vi "KCubeActionEngine.vi"(5 "ChannelNumber":i32, 7 "Position Settings":T2={"Step Size (mm)"=10.0, "Initial Position"=0.0, "Num Of Steps"=200, "Move Position"=0.0, "Step Delay (ms)"=0} {"Step Size (mm)" min=0.00046 format="%.8f"}, 8 "SerialNumber":string="26004239", 9 "KCubeStepperControl":refnum<k24>(container), 10 "Action":T3) -> (0 "error out":errorcluster, 2 "Current Position":dbl)   [LabVIEW 2022 SP3]
uses:
  C:/Users/ulate/Documents/mnOP/mnOPSuite-main/PRISM/Thorlabs.MotionControl.Controls.dll
  mnOPSuite-main/PRISM/Thorlabs.MotionControl.Controls.dll
  ActionEngineEnum.ctl
  C:/Users/ulate/Documents/mnOP/mnOPSuite-main/PRISM/Thorlabs.MotionControl.KCube.StepperMotorCLI.dll
  mnOPSuite-main/PRISM/Thorlabs.MotionControl.KCube.StepperMotorCLI.dll
  C:/Users/ulate/Documents/mnOP/mnOPSuite-main/PRISM/Thorlabs.MotionControl.GenericMotorCLI.dll
  mnOPSuite-main/PRISM/Thorlabs.MotionControl.GenericMotorCLI.dll
panel:
  out "DeviceSettingsBasedOnName":string
  in  "startupSettingsMode":i32(ring)=1 items=["UseDeviceSettings"=1, "UseFileSettings"=2, "UseConfiguredSettings"=3]
  out "Settings":T1
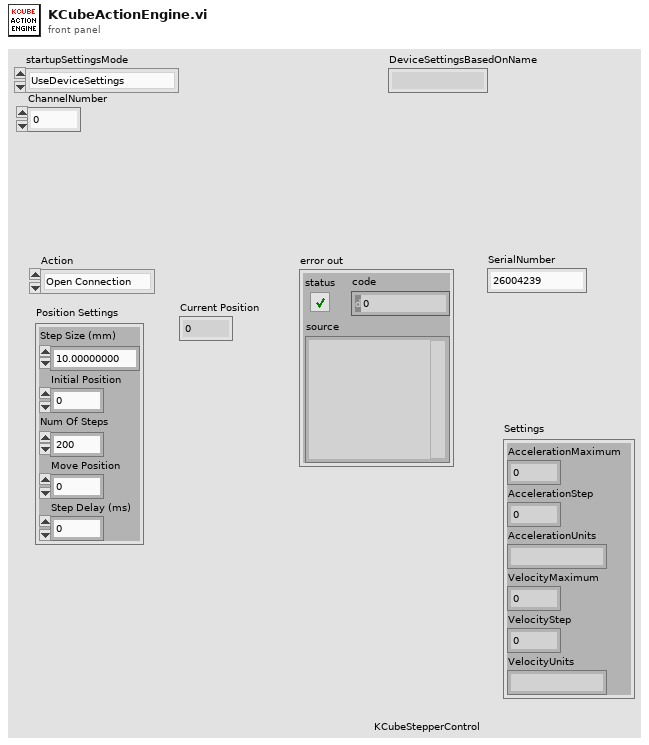
[diagram p1: front panel]
types:
  T1 = cluster{"AccelerationMaximum":dbl, "AccelerationStep":dbl, "AccelerationUnits":string, "VelocityMaximum":dbl, "VelocityStep":dbl, "VelocityUnits":string}
  T2 = cluster{"Step Size (mm)":sgl, "Initial Position":dbl, "Num Of Steps":i32, "Move Position":dbl, "Step Delay (ms)":u32}
  T3 = typedef "ActionEngineEnum.ctl" = enum16{"Open Connection", "Done", "Get Position", "Settings", "Home", "Move Absolute", "Move Relative", "Step", "Close Connection"}
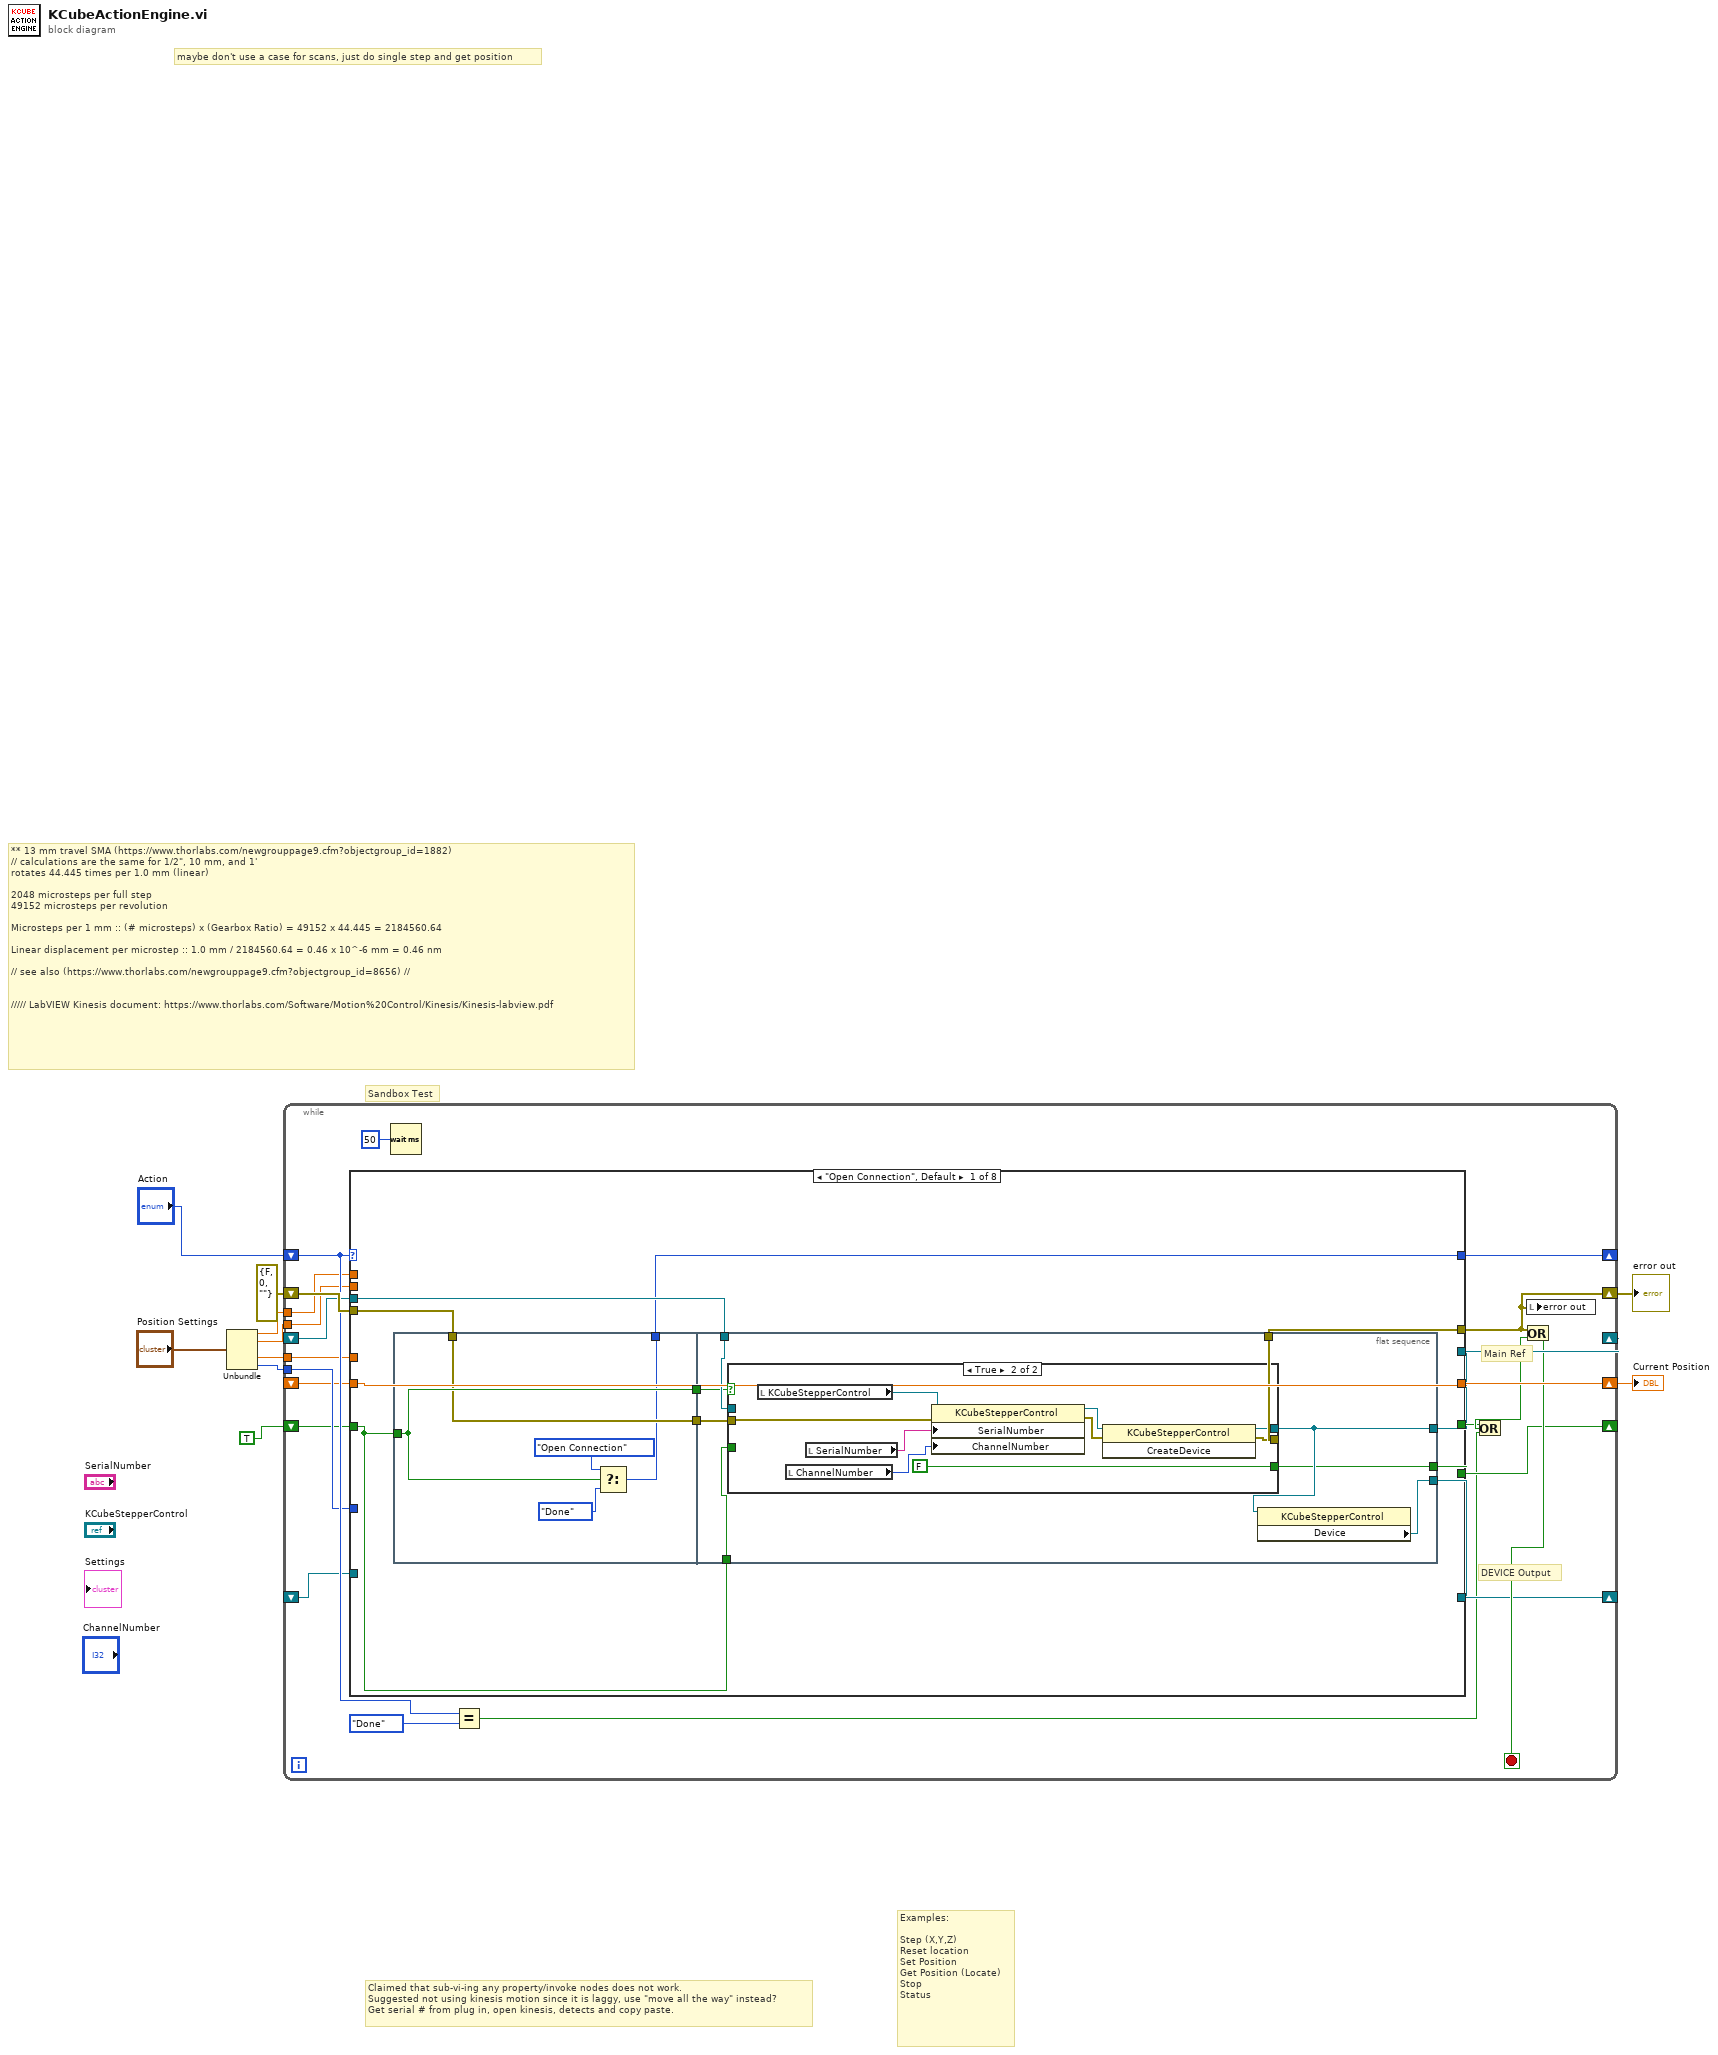
[diagram p0: block diagram]
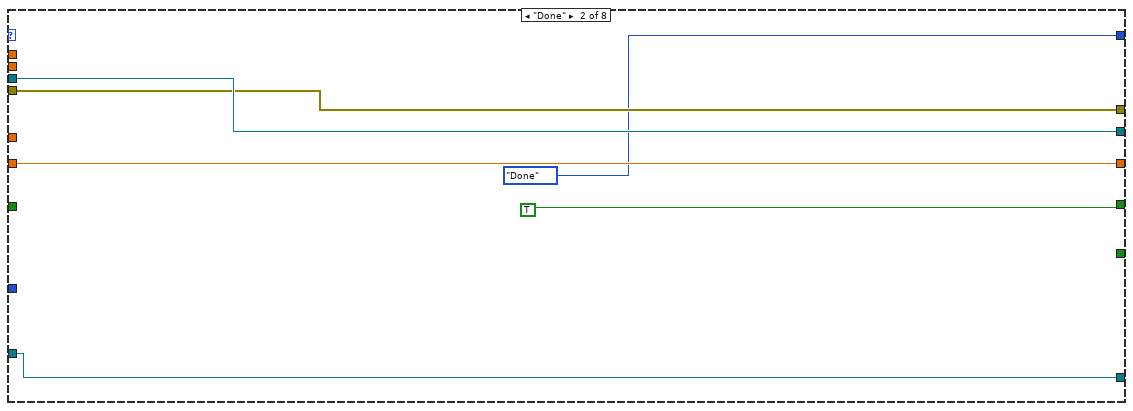
[diagram p3: hidden frame]
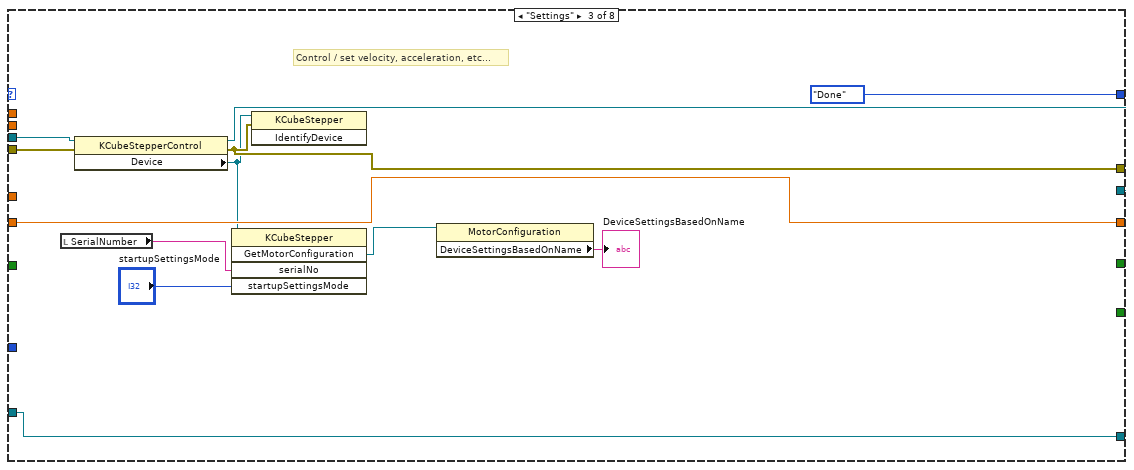
[diagram p4: hidden frame]
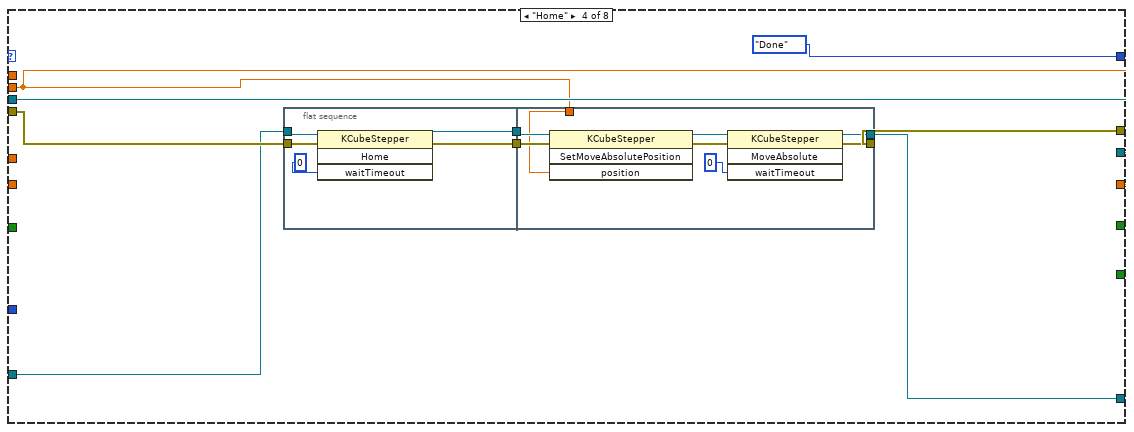
[diagram p5: hidden frame]
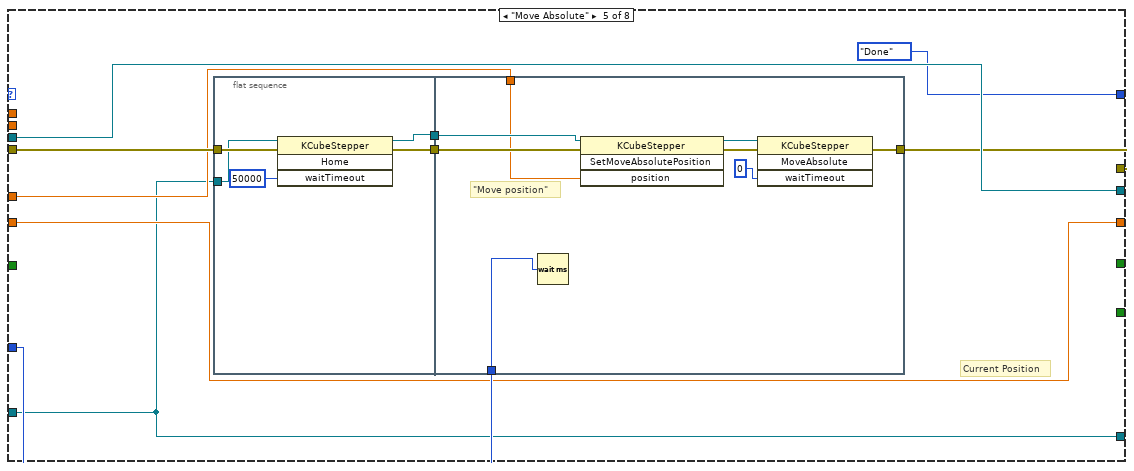
[diagram p6: hidden frame]
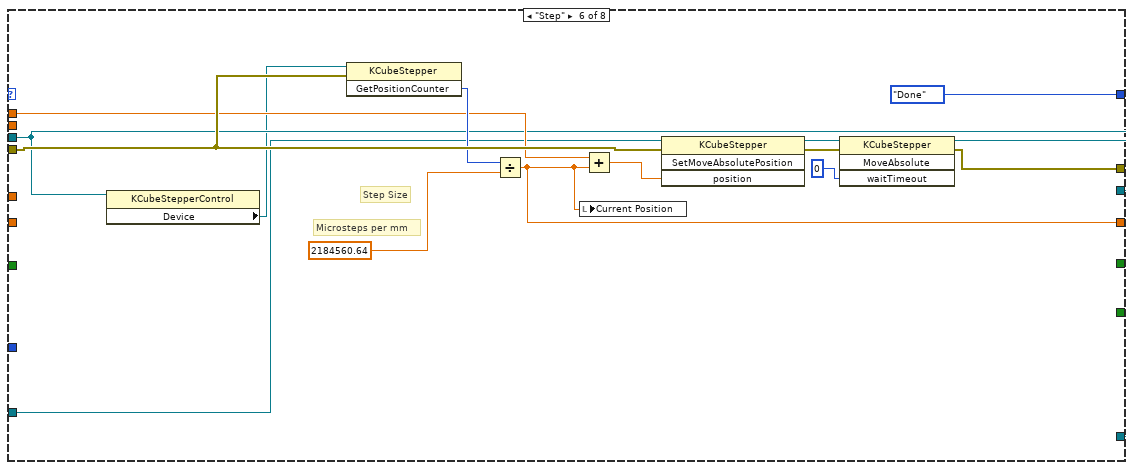
[diagram p7: hidden frame]
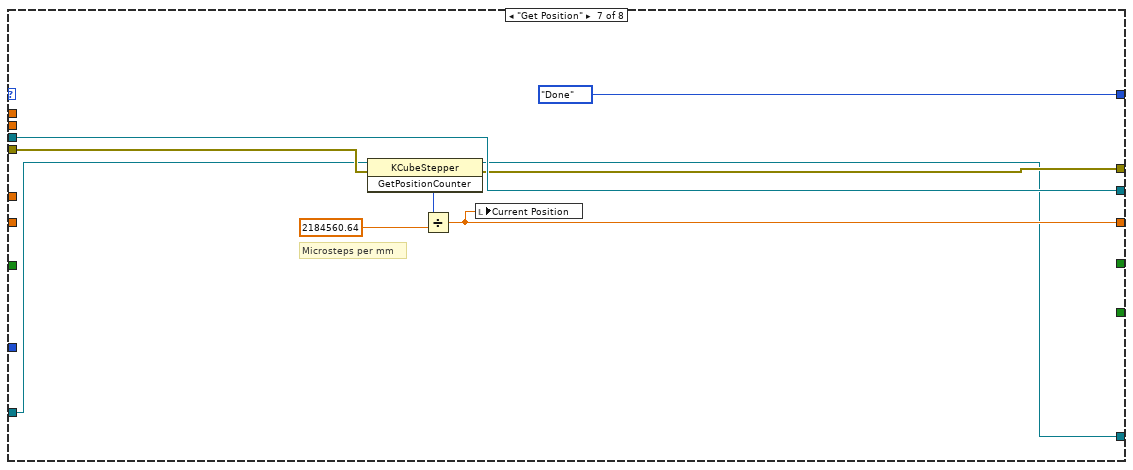
[diagram p8: hidden frame]
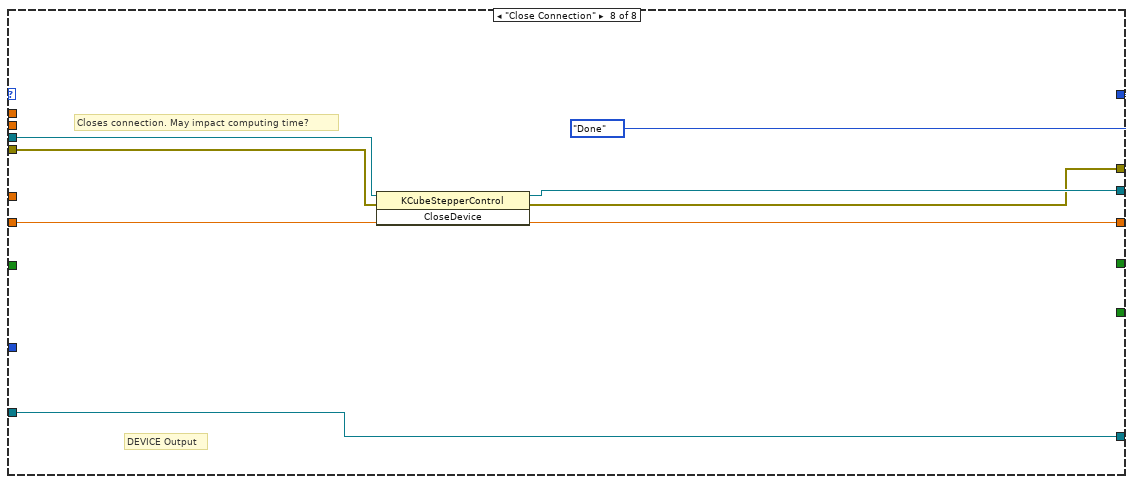
[diagram p9: hidden frame]
diagram:
  # "Claimed that sub-vi-ing any property/invoke nodes does not work.\nSuggested not using kinesis motion since it is laggy, use \"move all the way\" instead?\nGet serial # from plug in, open kinesis, detects and copy paste."
  # "maybe don't use a case for scans, just do single step and get position"
  # "Examples:\n\nStep (X,Y,Z)\nReset location\nSet Position\nGet Position (Locate) \nStop\nStatus"
  # "** 13 mm travel SMA (https://www.thorlabs.com/newgrouppage9.cfm?objectgroup_id=1882)\n// calculations are the same for 1/2\", 10 mm, and 1'\nrotates 44.445 times per 1.0 mm (linear)\n\n2048 microsteps per full step\n49152 microsteps per revolution\n\nMicrosteps per 1 mm :: (# microsteps) x (Gearbox Ratio) = 49152 x 44.445 = 2184560.64\n\nLinear displacement per microstep :: 1.0 mm / 2184560.64 = 0.46 x 10^-6 mm = 0.46 nm\n\n// see also (https://www.thorlabs.com/newgrouppage9.cfm?objectgroup_id=8656) //\n\n\n///// LabVIEW Kinesis document: https://www.thorlabs.com/Software/Motion%20Control/Kinesis/Kinesis-labview.pdf"
  # "Sandbox Test"
  n1 = Unbundle("Position Settings") -> ("Step Size (mm)"=w7:sgl, "Initial Position"=w8:dbl, "Move Position"=w5:dbl, "Step Delay (ms)"=w6:u32)  [unwired: 1 out]
  n2 = while {
    shift-right: [w19] -> w10
    shift-left: errorcluster {"status"=FALSE, "code"=0, "source"=""} ("error out") -> [w32]
    shift-right: [w30] -> _
    shift-left: _ -> [w31]
    shift-right: [w28] -> _
    shift-left: "Action" -> [w29]
    tunnel: w8 -> [w25]
    tunnel: w7 -> [w24]
    tunnel: w6 -> [w23]
    tunnel: w5 -> [w22]
    shift-right: [w21] -> w4
    shift-left: _ -> [w20]
    shift-right: [w17] -> _
    shift-left: _ -> [w16]
    shift-right: [w14] -> _
    shift-left: TRUE -> [w15]
    stop <- w18 stop-if-true
    # "DEVICE Output"
    # "Main Ref"
    n3 = case shown="\"Open Connection\", Default" w29 {
      tunnel: w32 -> [w42 w72 w84 w91 w118 w143 w154 w160]
      tunnel: [w39 w72 w81 w92 w110 w142 w151 w156] -> w19
      tunnel: w31 -> [w41 w73 w85 w95 w114 w133 w155 w158]
      tunnel: [w34 w73 w83 w95 w114 w133 w155 w157] -> w30
      tunnel: [w35 ActionEngineEnum."Done" ("Action") ActionEngineEnum."Done" ("Enum") ActionEngineEnum."Done" ("Enum") ActionEngineEnum."Done" ("Enum") ActionEngineEnum."Done" ("Enum") ActionEngineEnum."Done" ("Enum") ActionEngineEnum."Done" ("Enum")] -> w28
      tunnel: w25 -> [_ _ _ w90 _ _ _ _]
      tunnel: w24 -> [_ _ _ _ _ w138 _ _]
      tunnel: w23 -> [_ _ _ _ w115 _ _ _]
      tunnel: w22 -> [_ _ _ _ w113 _ _ _]
      tunnel: [w43 w74 w86 w90 w112 w137 w149 w161] -> w21
      tunnel: w20 -> [w43 w74 w86 _ w112 _ _ w161]
      tunnel: [w33 w71 w80 w88 w111 w135 w147 w159] -> w17
      tunnel: w16 -> [_ w71 w80 w89 w111 w134 w148 w159]
      tunnel: w15 -> [w40 _ _ _ _ _ _ _]
      tunnel: [w37 _ _ _ _ _ _ _] -> w14
      tunnel: [_ TRUE _ _ _ _ _ _] -> w11
      frame "Open Connection", Default {
        n4 = flat-sequence {
          tunnel: w40 -> [w48]
          tunnel: w42 -> [w45]
          tunnel: [w45] -> w38
          tunnel: [w48] -> w36
          tunnel: [w44] -> w35
          tunnel: w41 -> [w56]
          tunnel: w40 -> [w55]
          tunnel: [w49] -> w33
          tunnel: [w54] -> w39
          tunnel: [w52] -> w34
          tunnel: w38 -> [w53]
          tunnel: [w51] -> w37
          tunnel: w36 -> [w50]
          frame #0 {
            n5 = Select(t=ActionEngineEnum."Open Connection" ("Enum"), s=w48, f=ActionEngineEnum."Done" ("Enum")) -> (s? t:f=w44:T3)
          }
          frame #1 {
            n6 = case shown="True" w50 {
              selector: w50 -> [w57 _]
              tunnel: [w59 w66] -> w54
              tunnel: w53 -> [w59 w68]
              tunnel: [w58 w67] -> w52
              tunnel: w56 -> [w58 _]
              tunnel: w55 -> [_ _]
              tunnel: [w57 FALSE] -> w51
              frame False {
              }
              frame True {
                n7 = local read "KCubeStepperControl"() -> (w63:refnum<k24>)
                n8 = local read "ChannelNumber"() -> (w60:i32)
                n9 = local read "SerialNumber"() -> (w62:string)
                n10 = property class="KCubeStepperControl"(reference=w63, error in=w68, "SerialNumber"=w62, "ChannelNumber"=w60) -> (reference out=w65:refnum<k24>, error out=w64:errorcluster)
                n11 = invoke class="KCubeStepperControl" method="CreateDevice"(reference=w65, error in=w64) -> (reference out=w67:refnum<k24>, error out=w66:errorcluster)  [unwired: 1 in, 1 out]
              }
            }
            n12 = property class="KCubeStepperControl"(reference=w52) -> ("Device"=w49:refnum<k24>)  [unwired: 1 in, 2 out]
          }
        }
      }
      frame "Done" {
      }
      frame "Settings" {
        # "Control / set velocity, acceleration, etc..."
        n13 = local read "SerialNumber"() -> (w78:string)
        n14 = property class="KCubeStepperControl"(reference=w85, error in=w84) -> (reference out=w83:refnum<k24>, error out=w81:errorcluster, "Device"=w76:refnum<k24>)
        n15 = invoke class="KCubeStepper" method="GetMotorConfiguration"(reference=w76, "serialNo"=w78, "startupSettingsMode"="startupSettingsMode") -> ("GetMotorConfiguration"=w75:refnum<k24>)  [unwired: 2 in, 4 out]
        n16 = invoke class="KCubeStepper" method="IdentifyDevice"(reference=w76, error in=w81) -> ()  [unwired: 1 in, 3 out]
        n17 = property class="MotorConfiguration"(reference=w75) -> ("DeviceSettingsBasedOnName"=→"DeviceSettingsBasedOnName":string)  [unwired: 1 in, 2 out]
      }
      frame "Home" {
        n18 = flat-sequence {
          tunnel: w89 -> [w100]
          tunnel: w91 -> [w98]
          tunnel: [w97] -> w94
          tunnel: [w96] -> w93
          tunnel: w94 -> [w108]
          tunnel: w93 -> [w107]
          tunnel: [w103] -> w92
          tunnel: w90 -> [w102]
          tunnel: [w101] -> w88
          frame #0 {
            n19 = invoke class="KCubeStepper" method="Home"(reference=w100, error in=w98, "waitTimeout"=0) -> (reference out=w97:refnum<k24>, error out=w96:errorcluster)  [unwired: 1 in, 2 out]
          }
          frame #1 {
            n20 = invoke class="KCubeStepper" method="SetMoveAbsolutePosition"(reference=w108, error in=w107, "position"=w102) -> (reference out=w105:refnum<k24>, error out=w106:errorcluster)  [unwired: 1 in, 2 out]
            n21 = invoke class="KCubeStepper" method="MoveAbsolute"(reference=w105, error in=w106, "waitTimeout"=0) -> (reference out=w101:refnum<k24>, error out=w103:errorcluster)  [unwired: 1 in, 2 out]
          }
        }
      }
      frame "Move Absolute" {
        # "Current Position"
        n22 = flat-sequence {
          tunnel: w111 -> [w119]
          tunnel: w118 -> [w120]
          tunnel: [w122] -> w117
          tunnel: [w121] -> w116
          tunnel: w117 -> [w131]
          tunnel: w116 -> [w130]
          tunnel: [w129] -> w110
          tunnel: w115 -> [w128]
          tunnel: w113 -> [w124]
          frame #0 {
            n23 = invoke class="KCubeStepper" method="Home"(reference=w119, error in=w120, "waitTimeout"=50000) -> (reference out=w122:refnum<k24>, error out=w121:errorcluster)  [unwired: 1 in, 2 out]
          }
          frame #1 {
            # "\"Move position\""
            n24 = Wait (ms)(milliseconds to wait=w128) -> ()  [unwired: 1 out]
            n25 = invoke class="KCubeStepper" method="SetMoveAbsolutePosition"(reference=w131, error in=w130, "position"=w124) -> (reference out=w126:refnum<k24>, error out=w127:errorcluster)  [unwired: 1 in, 2 out]
            n26 = invoke class="KCubeStepper" method="MoveAbsolute"(reference=w126, error in=w127, "waitTimeout"=0) -> (error out=w129:errorcluster)  [unwired: 1 in, 3 out]
          }
        }
      }
      frame "Step" {
        # "Step Size"
        # "Microsteps per mm"
        n27 = property class="KCubeStepperControl"(reference=w133) -> ("Device"=w132:refnum<k24>)  [unwired: 1 in, 2 out]
        n28 = invoke class="KCubeStepper" method="GetPositionCounter"(reference=w132, error in=w143) -> ("GetPositionCounter"=w141:i32)  [unwired: 1 in, 2 out]
        n29 = Divide(x=w141, y=2184560.64) -> (x/y=w137:dbl)
        n30 = local write "Current Position"(w137) -> ()
        n31 = Add(x=w138, y=w137) -> (x+y=w139:dbl)
        n32 = invoke class="KCubeStepper" method="SetMoveAbsolutePosition"(reference=w134, error in=w143, "position"=w139) -> (reference out=w145:refnum<k24>, error out=w146:errorcluster)  [unwired: 1 in, 2 out]
        n33 = invoke class="KCubeStepper" method="MoveAbsolute"(reference=w145, error in=w146, "waitTimeout"=0) -> (reference out=w135:refnum<k24>, error out=w142:errorcluster)  [unwired: 1 in, 2 out]
      }
      frame "Get Position" {
        # "Microsteps per mm"
        n34 = invoke class="KCubeStepper" method="GetPositionCounter"(reference=w148, error in=w154) -> (reference out=w147:refnum<k24>, error out=w151:errorcluster, "GetPositionCounter"=w153:i32)  [unwired: 1 in]
        n35 = Divide(x=w153, y=2184560.64) -> (x/y=w149:dbl)
        n36 = local write "Current Position"(w149) -> ()
      }
      frame "Close Connection" {
        # "DEVICE Output"
        # "Closes connection. May impact computing time?"
        n37 = invoke class="KCubeStepperControl" method="CloseDevice"(reference=w158, error in=w160) -> (reference out=w157:refnum<k24>, error out=w156:errorcluster)  [unwired: 1 in, 1 out]
      }
    }
    n38 = Wait (ms)(milliseconds to wait=u32 50) -> ()  [unwired: 1 out]
    n39 = Equal?(x=w29, y=ActionEngineEnum."Done" ("Enum")) -> (x = y?=w12:bool)
    n40 = Or(x=w11, y=w12) -> (x .or. y?=w13:bool)
    n41 = Or(x=w19, y=w13) -> (x .or. y?=w18:bool)
    n42 = local write "error out"(w19) -> ()
  }
  "error out" <- w10
  "Current Position" <- w4
